vi "Configure List Termination Value.vi"(8 "error in (no error)":errorcluster, 9 "Termination Value (0: Before List Starting Value)":i32(ring) items=["Before List Starting Value", "Last Step Value"], 10 "Channel (1)":string="1", 11 "VISA resource name":refnum<visa-resource-name>) -> (0 "error out":errorcluster, 3 "VISA resource name out":refnum<visa-resource-name>)   [LabVIEW 2020, in "Keysight E36300 Series.lvlib"]
doc: "Configures the list termination value.\n\n<b>Note: </b>\nThis VI is only applicable for E36312A and E36313A models."
uses:
  Keysight E36300 Series.lvlib
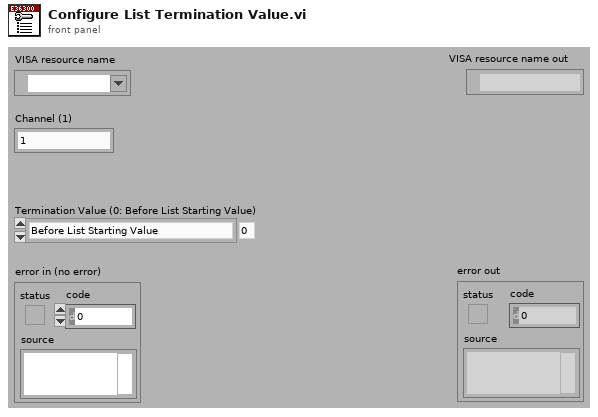
[diagram p1: front panel]
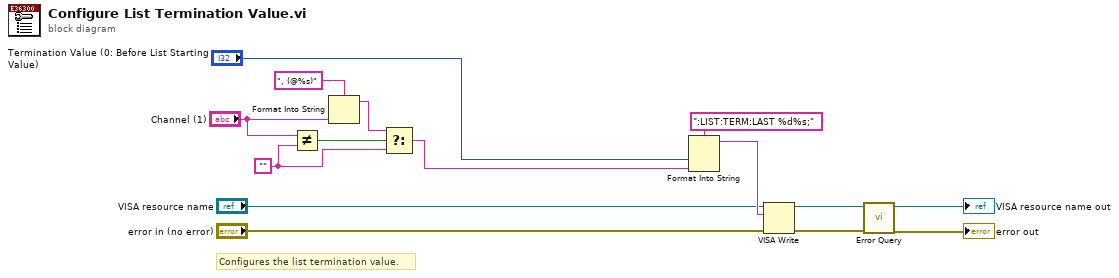
[diagram p0: block diagram]
diagram:
  w1 = ""
  # "Configures the list termination value."
  n1 = Not Equal?(x="Channel (1)", y=w1) -> (x != y?=w4:bool)
  n2 = Format Into String(format string=", (@%s)", "Channel (1)") -> (resulting string=w5:string)  [unwired: 2 in, 1 out]
  n3 = Select(t=w5, s=w4, f=w1) -> (s? t:f=w2:string)
  n4 = Format Into String(format string=":LIST:TERM:LAST %d%s;", "Termination Value (0: Before List Starting Value)", w2) -> (resulting string=w13:string)  [unwired: 2 in, 1 out]
  n5 = VISA Write(VISA resource name="VISA resource name", write buffer=w13, error in (no error)="error in (no error)") -> (VISA resource name out=w10:refnum<visa-resource-name>, error out=w9:errorcluster)  [unwired: 1 out]
  n6 = call "Error Query.vi"("error in (no error)"=w9, "VISA resource name"=w10) -> ("error out"=→"error out":errorcluster, "VISA resource name out"=→"VISA resource name out":refnum<visa-resource-name>)  [unwired: 6 in, 2 out]
